vi "check.vi"(8 "action list IN":refnum<class "action.lvclass">[](array[class]), 9 "action IN":refnum<class "action.lvclass">, 11 "action stack In":refnum<class "action.lvclass">[](array[class])) -> (1 "action OUT":refnum<class "action.lvclass">, 2 "stack is empty ?":bool, 3 "action stack Out":refnum<class "action.lvclass">[](array[class]))   [LabVIEW 2018, in "action.lvclass"]
uses:
  action.lvclass
  stack action -- control.ctl
  action.lvclass/action.ctl
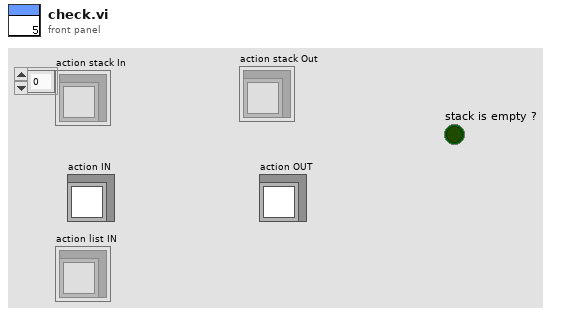
[diagram p1: front panel]
types:
  T1 = typedef "stack action -- control.ctl" = enum16{"push", "pop", "check", "init"}
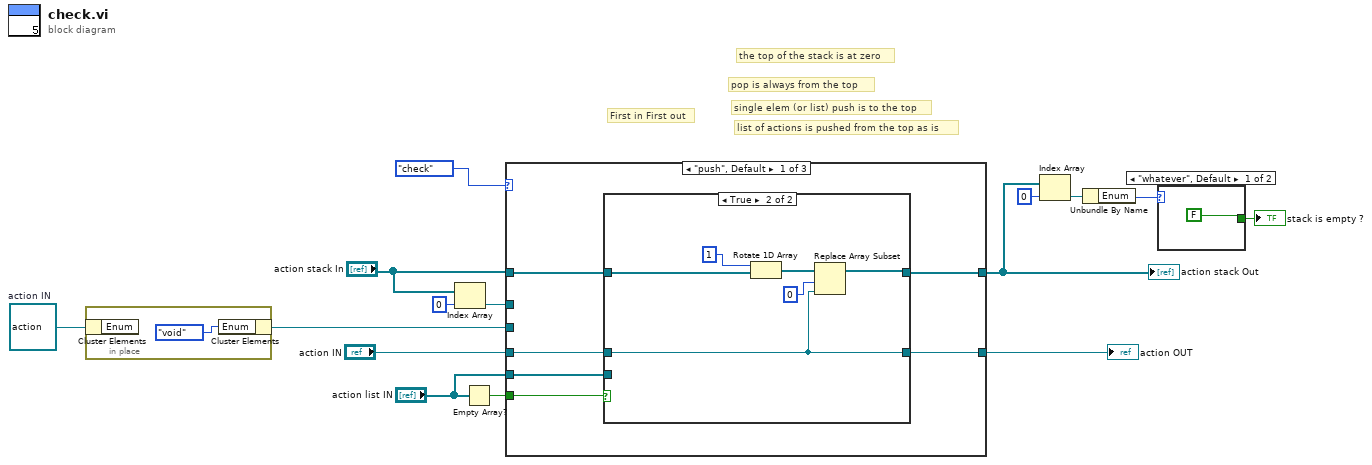
[diagram p0: block diagram]
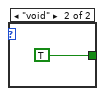
[diagram p2: hidden frame]
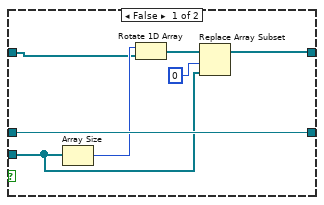
[diagram p3: hidden frame]
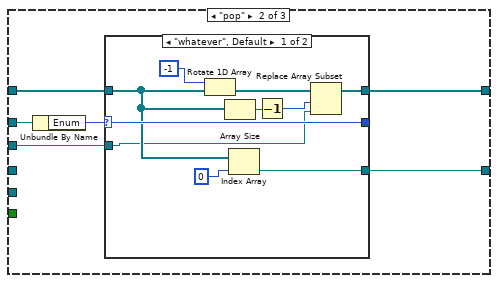
[diagram p4: hidden frame]
diagram:
  w4 = refnum<class "action.lvclass"> refnum  # action IN
  # "list of actions is pushed from the top as is"
  # "single elem (or list) push is to the top"
  # "pop is always from the top"
  # "First in First out"
  # "the top of the stack is at zero"
  n1 = in-place {
    n2 = in-place-cluster #1(w4) -> ()  [unwired: 1 out]
    n3 = in-place-cluster #1("Enum"=enum16{"void", "whatever"}."void") -> (w3:refnum<class "action.lvclass">)
  }
  n4 = Index Array(array="action stack In", index=0) -> (element=w12:refnum<class "action.lvclass">)
  n5 = Empty Array?(array="action list IN") -> (empty?=w14:bool)
  n6 = case shown="\"push\", Default" stack_action_--_control."check" ("stack action") {
    tunnel: [w22 w41 w55] -> w6
    tunnel: "action stack In" -> [w21 w40 w55]
    tunnel: w12 -> [_ w37 _]
    tunnel: [w17 w39 w56] -> w5
    tunnel: "action IN" -> [w20 _ w56]
    tunnel: w14 -> [w19 _ _]
    tunnel: "action list IN" -> [w18 _ _]
    tunnel: w3 -> [_ w38 _]
    frame "push", Default {
      n7 = case shown="True" w19 {
        tunnel: [w23 w31] -> w22
        tunnel: w21 -> [w27 w33]
        tunnel: w20 -> [w29 w30]
        tunnel: w18 -> [w24 _]
        tunnel: [w29 w30] -> w17
        frame False {
          n8 = Array Size(array=w24) -> (size(s)=w28:i32)
          n9 = Rotate 1D Array(1:w27, 2:w28) -> (0:w26:refnum<class "action.lvclass">[])
          n10 = Replace Array Subset(array=w26, new element=w24, index=0) -> (w23:refnum<class "action.lvclass">[])
        }
        frame True {
          n11 = Rotate 1D Array(1:w33, 2:1) -> (0:w35:refnum<class "action.lvclass">[])
          n12 = Replace Array Subset(array=w35, new element=w30, index=0) -> (w31:refnum<class "action.lvclass">[])
        }
      }
    }
    frame "pop" {
      n13 = Unbundle By Name(w37) -> ("Enum"=w36:enum16{"void", "whatever"})
      n14 = case shown="\"whatever\", Default" w36 {
        selector: w36 -> [w49 w53]
        tunnel: [w45 w54] -> w41
        tunnel: w40 -> [w46 w54]
        tunnel: [w50 w52] -> w39
        tunnel: [w49 w53] -> _
        tunnel: w38 -> [w42 w52]
        frame "whatever", Default {
          n15 = Rotate 1D Array(1:w46, 2:-1) -> (0:w44:refnum<class "action.lvclass">[])
          n16 = Array Size(array=w46) -> (size(s)=w47:i32)
          n17 = Index Array(array=w46, index=0) -> (element=w50:refnum<class "action.lvclass">)
          n18 = Decrement(x=w47) -> (x-1=w43:i32)
          n19 = Replace Array Subset(array=w44, new element=w42, index=w43) -> (w45:refnum<class "action.lvclass">[])
        }
        frame "void" {
        }
      }
    }
    frame "check" {
    }
  }
  "action stack Out" <- w6
  "action OUT" <- w5
  n20 = Index Array(array=w6, index=0) -> (element=w2:refnum<class "action.lvclass">)
  n21 = Unbundle By Name(w2) -> ("Enum"=w1:enum16{"void", "whatever"})
  n22 = case shown="\"whatever\", Default" w1 {
    tunnel: [FALSE TRUE] -> w10
    frame "whatever", Default {
    }
    frame "void" {
    }
  }
  "stack is empty ?" <- w10
